vi "Flatten UIP Value.vi"(11 "UIP In":refnum<class "DescriptionUIP.lvclass">) -> (0 "Error Out":errorcluster, 2 "String Value":string, 3 "UIP Out":refnum<class "DescriptionUIP.lvclass">)   [LabVIEW 2015, in "DescriptionUIP.lvclass"]
uses:
  DescriptionUIP.lvclass
  DescriptionUIP.lvclass/DescriptionUIP.ctl
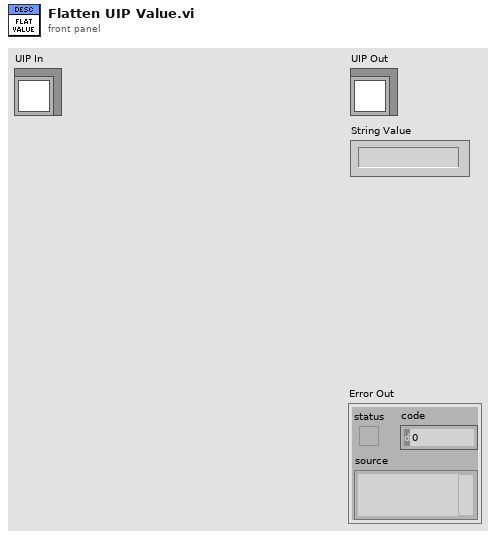
[diagram p1: front panel]
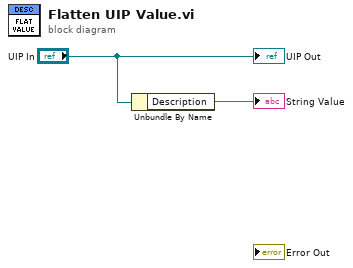
[diagram p0: block diagram]
diagram:
  n1 = Unbundle By Name("UIP In") -> ("Description"=→"String Value":string)
  "UIP Out" <- "UIP In"
